vi "parseMOCONstring.vi"(11 "MOCONstring":string="2021/07/19\t13:21:53\t4.219\tppm\t \t \t40.1\t34.9\t177.2\t1.1560e-10\t2.623460e+05\t-2.610868e-05\t65.09\r\n") -> (2 "channelsArray":dbl[](array[numeric]))   [LabVIEW 2020]
uses:
  <vilib>/Utility/miscctls.llb/LVDateTimeRec.ctl
panel:
  out "temperature(ch13)":dbl
  out "detectorCurrent(ch10)":dbl
  out "airFlow(ch9)":dbl
  out "fuelFlow(ch8)":dbl
  out "sampFlow(ch7)":dbl
  out "Conc(ch3)":dbl
  out "timestamp(ch0)":dbl
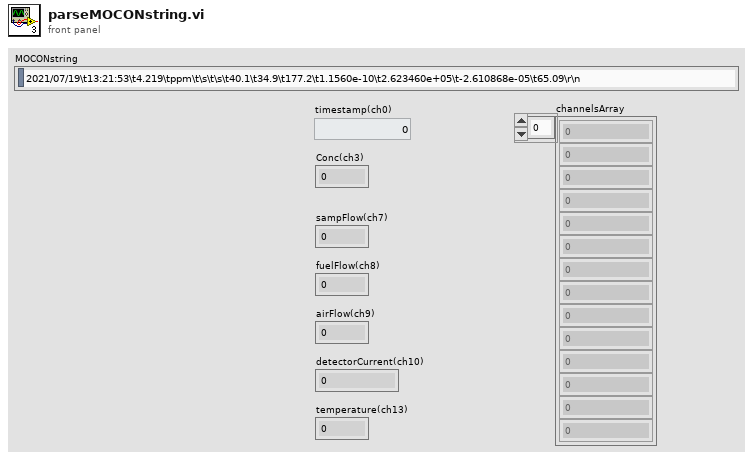
[diagram p1: front panel]
types:
  T1 = typedef "LVDateTimeRec.ctl" = cluster{"fractional second":dbl, "second":i32, "minute":i32, "hour":i32, "day of month":i32, "month":i32, "year":i32, "day of week":i32, "day of year":i32, "DST":i32}
  T2 = cluster{"[0]":string, "[1]":string, "[2]":string, "[3]":string, "[4]":string, "[5]":string, "[6]":string, "[7]":string, "[8]":string, "[9]":string, "[10]":string, "[11]":string, "[12]":string}
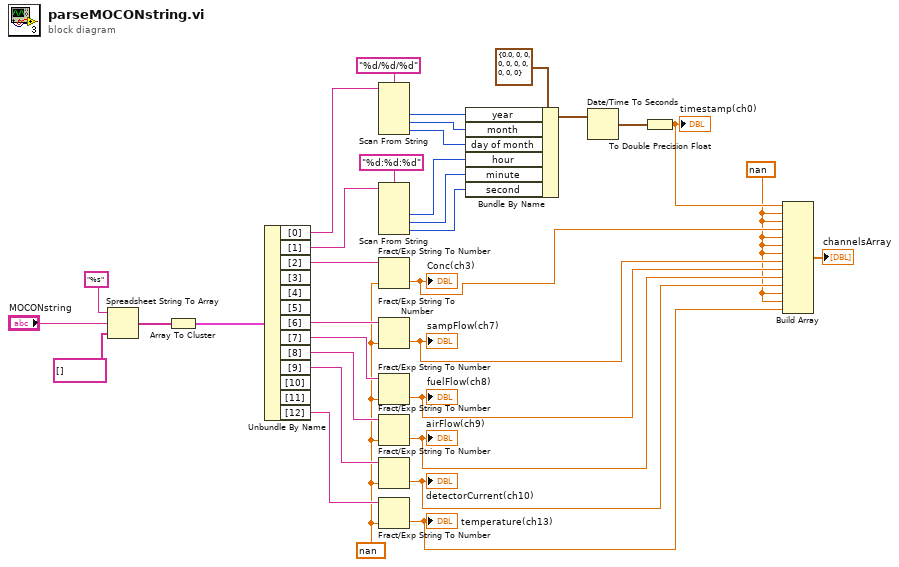
[diagram p0: block diagram]
diagram:
  w1 = nan
  w4 = nan
  n1 = Spreadsheet String To Array(format string="%s", spreadsheet string="MOCONstring", array type (2D Dbl)=string[] []) -> (array=w31:string[])  [unwired: 1 in]
  n2 = Array To Cluster(array=w31) -> (cluster=w30:T2)
  n3 = Unbundle By Name(w30) -> ("[0]"=w25:string, "[1]"=w20:string, "[2]"=w29:string, "[6]"=w15:string, "[7]"=w12:string, "[8]"=w11:string, "[9]"=w13:string, "[12]"=w14:string)  [unwired: 5 out]
  n4 = Scan From String(format string="%d/%d/%d", input string=w25) -> (output 1=w23:i32, output 2=w22:i32, output 3=w21:i32)  [unwired: 5 in, 3 out]
  n5 = Scan From String(format string="%d:%d:%d", input string=w20) -> (output 1=w18:i32, output 2=w17:i32, output 3=w16:i32)  [unwired: 5 in, 3 out]
  n6 = Fract/Exp String To Number(string=w29, default (0 dbl)=w1) -> (number=w9:dbl)  [unwired: 2 in, 1 out]
  "Conc(ch3)" <- w9
  n7 = Fract/Exp String To Number(string=w15, default (0 dbl)=w1) -> (number=w8:dbl)  [unwired: 2 in, 1 out]
  "sampFlow(ch7)" <- w8
  n8 = Fract/Exp String To Number(string=w12, default (0 dbl)=w1) -> (number=w7:dbl)  [unwired: 2 in, 1 out]
  "fuelFlow(ch8)" <- w7
  n9 = Fract/Exp String To Number(string=w11, default (0 dbl)=w1) -> (number=w6:dbl)  [unwired: 2 in, 1 out]
  "airFlow(ch9)" <- w6
  n10 = Fract/Exp String To Number(string=w13, default (0 dbl)=w1) -> (number=w5:dbl)  [unwired: 2 in, 1 out]
  "detectorCurrent(ch10)" <- w5
  n11 = Fract/Exp String To Number(string=w14, default (0 dbl)=w1) -> (number=w3:dbl)  [unwired: 2 in, 1 out]
  "temperature(ch13)" <- w3
  n12 = Bundle By Name(cluster=T1 {"fractional second"=0.0, "second"=0, "minute"=0, "hour"=0, "day of month"=0, "month"=0, "year"=0, "day of week"=0, "day of year"=0, "DST"=0} ("date time rec"), "year"=w23, "month"=w22, "day of month"=w21, "hour"=w18, "minute"=w17, "second"=w16) -> (w28:T1)
  n13 = Date/Time To Seconds(2:w28) -> (0:w26:timestamp)  [unwired: 1 in]
  n14 = To Double Precision Float(number=w26) -> (double precision float=w10:dbl)
  "timestamp(ch0)" <- w10
  n15 = Build Array(w10, w4, w4, w9, w4, w4, w4, w8, w7, w6, w5, w4, w4, w3) -> (→"channelsArray":dbl[])
